vi "GT Buf Jump Next Seg.vi"(6 "fifo":i16, 7 "limitType":i16, 8 "error in (no error)":errorcluster caption="错误输入（无错误）", 9 "axis":i16, 10 "crd":i16, 11 "cardNum":i16) -> (0 "error out":errorcluster caption="错误输出", 3 "function return":i16)   [LabVIEW 2014, in "gts.lvlib"]
doc: "GT_API GT_BufJumpNextSeg(short cardNum,short crd,short axis,short limitType,short fifo=0);"
uses:
  gts.lvlib
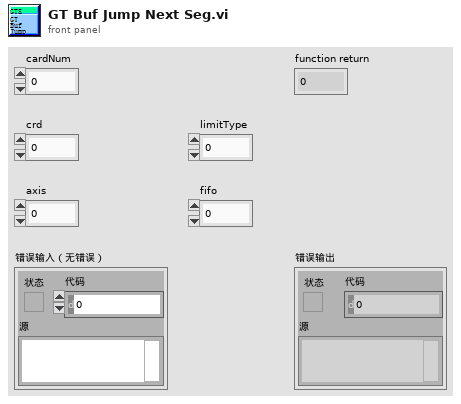
[diagram p1: front panel]
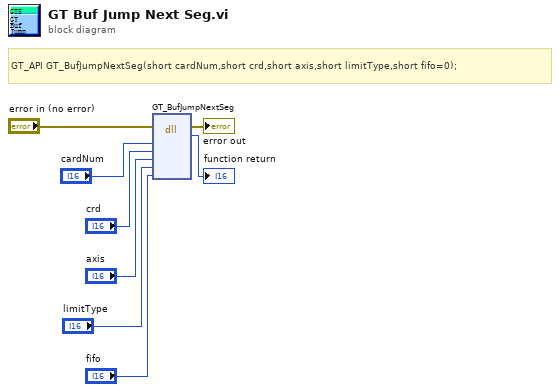
[diagram p0: block diagram]
diagram:
  # "GT_API GT_BufJumpNextSeg(short cardNum,short crd,short axis,short limitType,short fifo=0);"
  n1 = dll-call lib="PTH2habs D固高科技资料GTS控制卡GTS卡18年上半年资料dllVC32bit\nmulti_cardgts.*" fn="GT_BufJumpNextSeg"(error in="error in (no error)", "cardNum"="cardNum", "crd"="crd", "axis"="axis", "limitType"="limitType", "fifo"="fifo") -> (error out=→"error out":errorcluster, →"function return":i16)  [unwired: 7 in, 1 out]
